vi "qTNJ.vi"(0 "System no.":i32=1 min=1 max=4 step=1, 5 "error in":errorcluster) -> (14 "Number of Joysticks":i32, 19 "error out":errorcluster)   [LabVIEW 2026]
doc: "Returns the number of joysticks connected to the controller."
panel:
  # "Returns the number of joysticks connected to the controller."
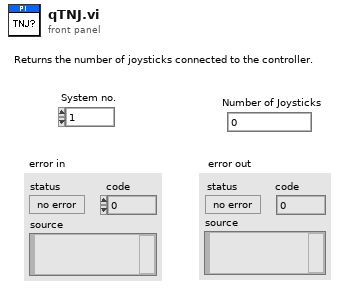
[diagram p1: front panel]
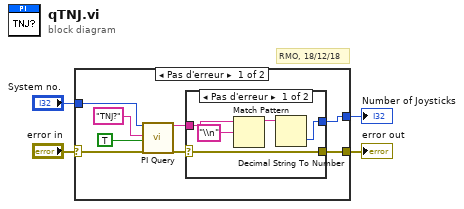
[diagram p0: block diagram]
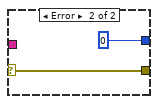
[diagram p2: hidden frame]
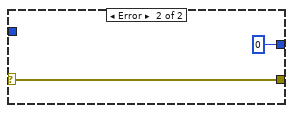
[diagram p3: hidden frame]
diagram:
  # "RMO, 18/12/18"
  n1 = case shown="Pas d'erreur" "error in" {
    selector: "error in" -> [w8 w21]
    tunnel: [w12 0] -> w4
    tunnel: [w5 w21] -> w3
    tunnel: "System no." -> [w10 _]
    frame No Error {
      n2 = call "PI Query.vi"("System no."=w10, "String to send"="TNJ?", "Attach termination char.?"=TRUE ("Attach Linefeed?"), "error in"=w8) -> ("String read"=w7:string, "error out"=w6:errorcluster)  [unwired: 3 in, 11 out]
      n3 = case shown="Pas d'erreur" w6 {
        selector: w6 -> [w13 w18]
        tunnel: w7 -> [w16 _]
        tunnel: [w17 0] -> w12
        tunnel: [w13 w18] -> w5
        frame No Error {
          n4 = Match Pattern(string=w16, regular expression="\\n") -> (before substring=w14:string)  [unwired: 4 out]
          n5 = Decimal String To Number(string=w14) -> (number=w17:i32)  [unwired: 3 out]
        }
        frame Error {
        }
      }
    }
    frame Error {
    }
  }
  "error out" <- w3
  "Number of Joysticks" <- w4
